vi "u8_image.vi"(6 "non-flip":bool=TRUE, 7 "Enum":T1(ring), 9 "length":i32, 10 "index":i32, 11 "array":u8[](array[numeric])) -> (2 "Numeric":dbl, 3 "Array":dbl[](array[numeric]))   [LabVIEW 2014]
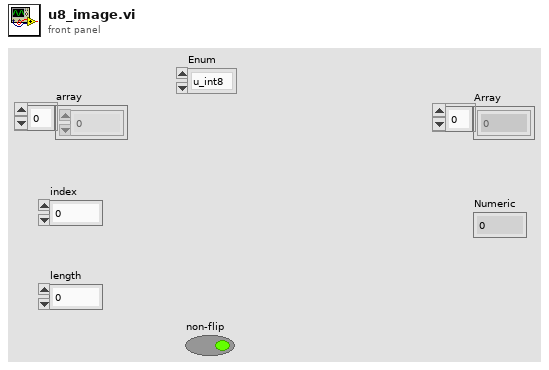
[diagram p1: front panel]
types:
  T1 = enum16{"u_int8", "int8", "u_int16", "int16", "u_int32", "int32", "u_int64", "int64", "float", "double"}
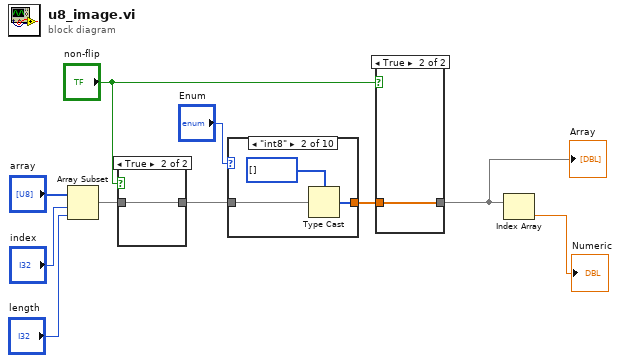
[diagram p0: block diagram]
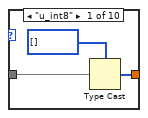
[diagram p2: hidden frame]
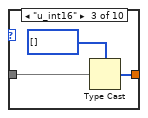
[diagram p3: hidden frame]
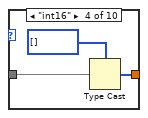
[diagram p4: hidden frame]
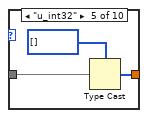
[diagram p5: hidden frame]
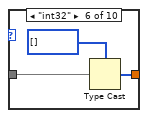
[diagram p6: hidden frame]
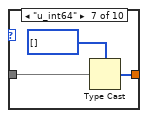
[diagram p7: hidden frame]
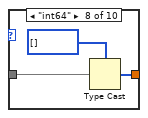
[diagram p8: hidden frame]
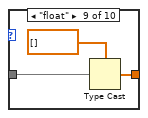
[diagram p9: hidden frame]
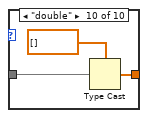
[diagram p10: hidden frame]
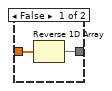
[diagram p11: hidden frame]
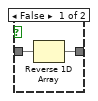
[diagram p12: hidden frame]
diagram:
  n1 = Array Subset(array="array", index="index", length="length") -> (w10:u8[])
  n2 = case shown="True" "non-flip" {
    tunnel: w10 -> [w12 w13]
    tunnel: [w11 w13] -> w4
    frame False {
      n3 = Reverse 1D Array(array=w12) -> (reversed array=w11:u8[])
    }
    frame True {
    }
  }
  n4 = case shown="\"int8\"" "Enum" {
    tunnel: [w14 w17 w20 w23 w26 w29 w32 w35 w38 w41] -> w2
    tunnel: w4 -> [w15 w18 w21 w24 w27 w30 w33 w36 w39 w42]
    frame "u_int8" {
      n5 = Type Cast(type=u8[] [], x=w15) -> (*(type *) &x=w14:u8[])
    }
    frame "int8" {
      n6 = Type Cast(type=i8[] [], x=w18) -> (*(type *) &x=w17:i8[])
    }
    frame "u_int16" {
      n7 = Type Cast(type=u16[] [], x=w21) -> (*(type *) &x=w20:u16[])
    }
    frame "int16" {
      n8 = Type Cast(type=i16[] [], x=w24) -> (*(type *) &x=w23:i16[])
    }
    frame "u_int32" {
      n9 = Type Cast(type=u32[] [], x=w27) -> (*(type *) &x=w26:u32[])
    }
    frame "int32" {
      n10 = Type Cast(type=i32[] [], x=w30) -> (*(type *) &x=w29:i32[])
    }
    frame "u_int64" {
      n11 = Type Cast(type=u64[] [], x=w33) -> (*(type *) &x=w32:u64[])
    }
    frame "int64" {
      n12 = Type Cast(type=i64[] [], x=w36) -> (*(type *) &x=w35:i64[])
    }
    frame "float" {
      n13 = Type Cast(type=sgl[] [], x=w39) -> (*(type *) &x=w38:sgl[])
    }
    frame "double" {
      n14 = Type Cast(type=dbl[] [], x=w42) -> (*(type *) &x=w41:dbl[])
    }
  }
  n15 = case shown="True" "non-flip" {
    tunnel: w2 -> [w45 w46]
    tunnel: [w44 w46] -> w1
    frame False {
      n16 = Reverse 1D Array(array=w45) -> (reversed array=w44:dbl[])
    }
    frame True {
    }
  }
  "Array" <- w1
  n17 = Index Array(array=w1) -> (element=→"Numeric":dbl)  [unwired: 1 in]
